vi "UI.vi"() -> ()   [LabVIEW 2017]
panel:
  in  "LoopBack Send":u16 format="%08b"
  out "Loopback Receive":u16 format="%08b"
  out "Results":dbl[](array[numeric])
  in  "Parameters":dbl[](array[numeric])
  out "Statusword":u16 format="%08b"
  in  "Controlword":u16 format="%08b"
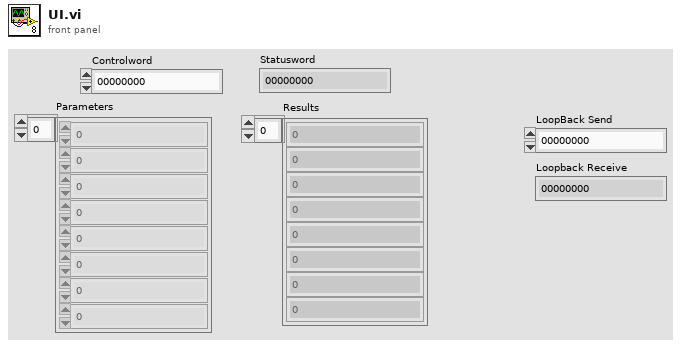
[diagram p1: front panel]
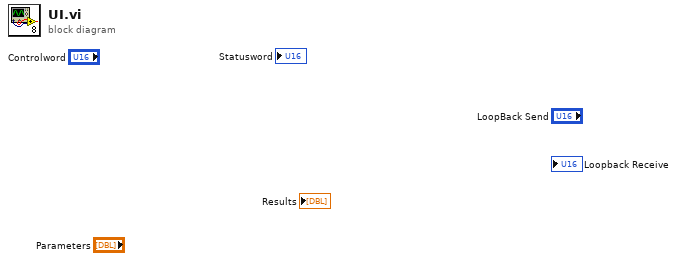
[diagram p0: block diagram]
diagram:
